vi "Save Editor Position to INI.vi"(8 "error in":errorcluster, 10 "Window Bounds":T1) -> (0 "error out":errorcluster)   [LabVIEW 2020, in "lv_icon.lvlib"]
doc: "Writes the position data to the LabVIEW INI file."
uses:
  lv_icon.lvlib
  <vilib>/Utility/miscctls.llb/LVRectTypeDef.ctl
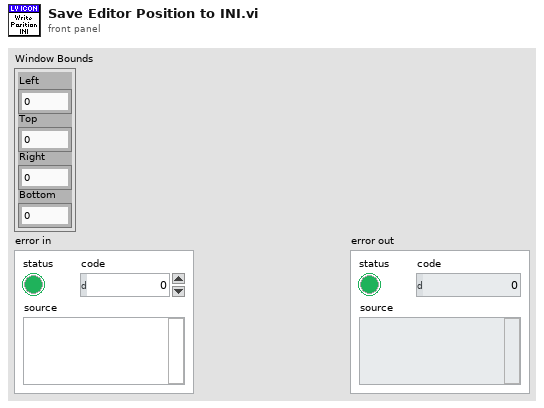
[diagram p1: front panel]
types:
  T1 = typedef "LVRectTypeDef.ctl" = cluster{"Left":i16, "Top":i16, "Right":i16, "Bottom":i16}
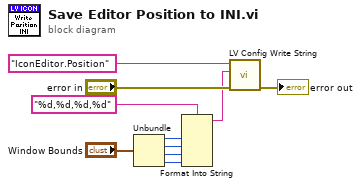
[diagram p0: block diagram]
diagram:
  n1 = Unbundle("Window Bounds") -> ("Left"=w8:i16, "Top"=w7:i16, "Right"=w6:i16, "Bottom"=w5:i16)
  n2 = Format Into String(format string="%d,%d,%d,%d", w8, w7, w6, w5) -> (resulting string=w3:string)  [unwired: 2 in, 1 out]
  n3 = call <resource>:"LV Config Write String.vi"("error in (no error)"="error in", "value"=w3, "key"="IconEditor.Position") -> ("error out"=→"error out":errorcluster)  [unwired: 4 in]
